vi "A14rowin.vi"(11 "Basic Size":ext) -> (3 "Row":ext)   [LabVIEW 2023]
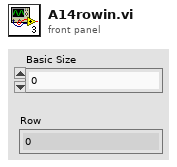
[diagram p1: front panel]
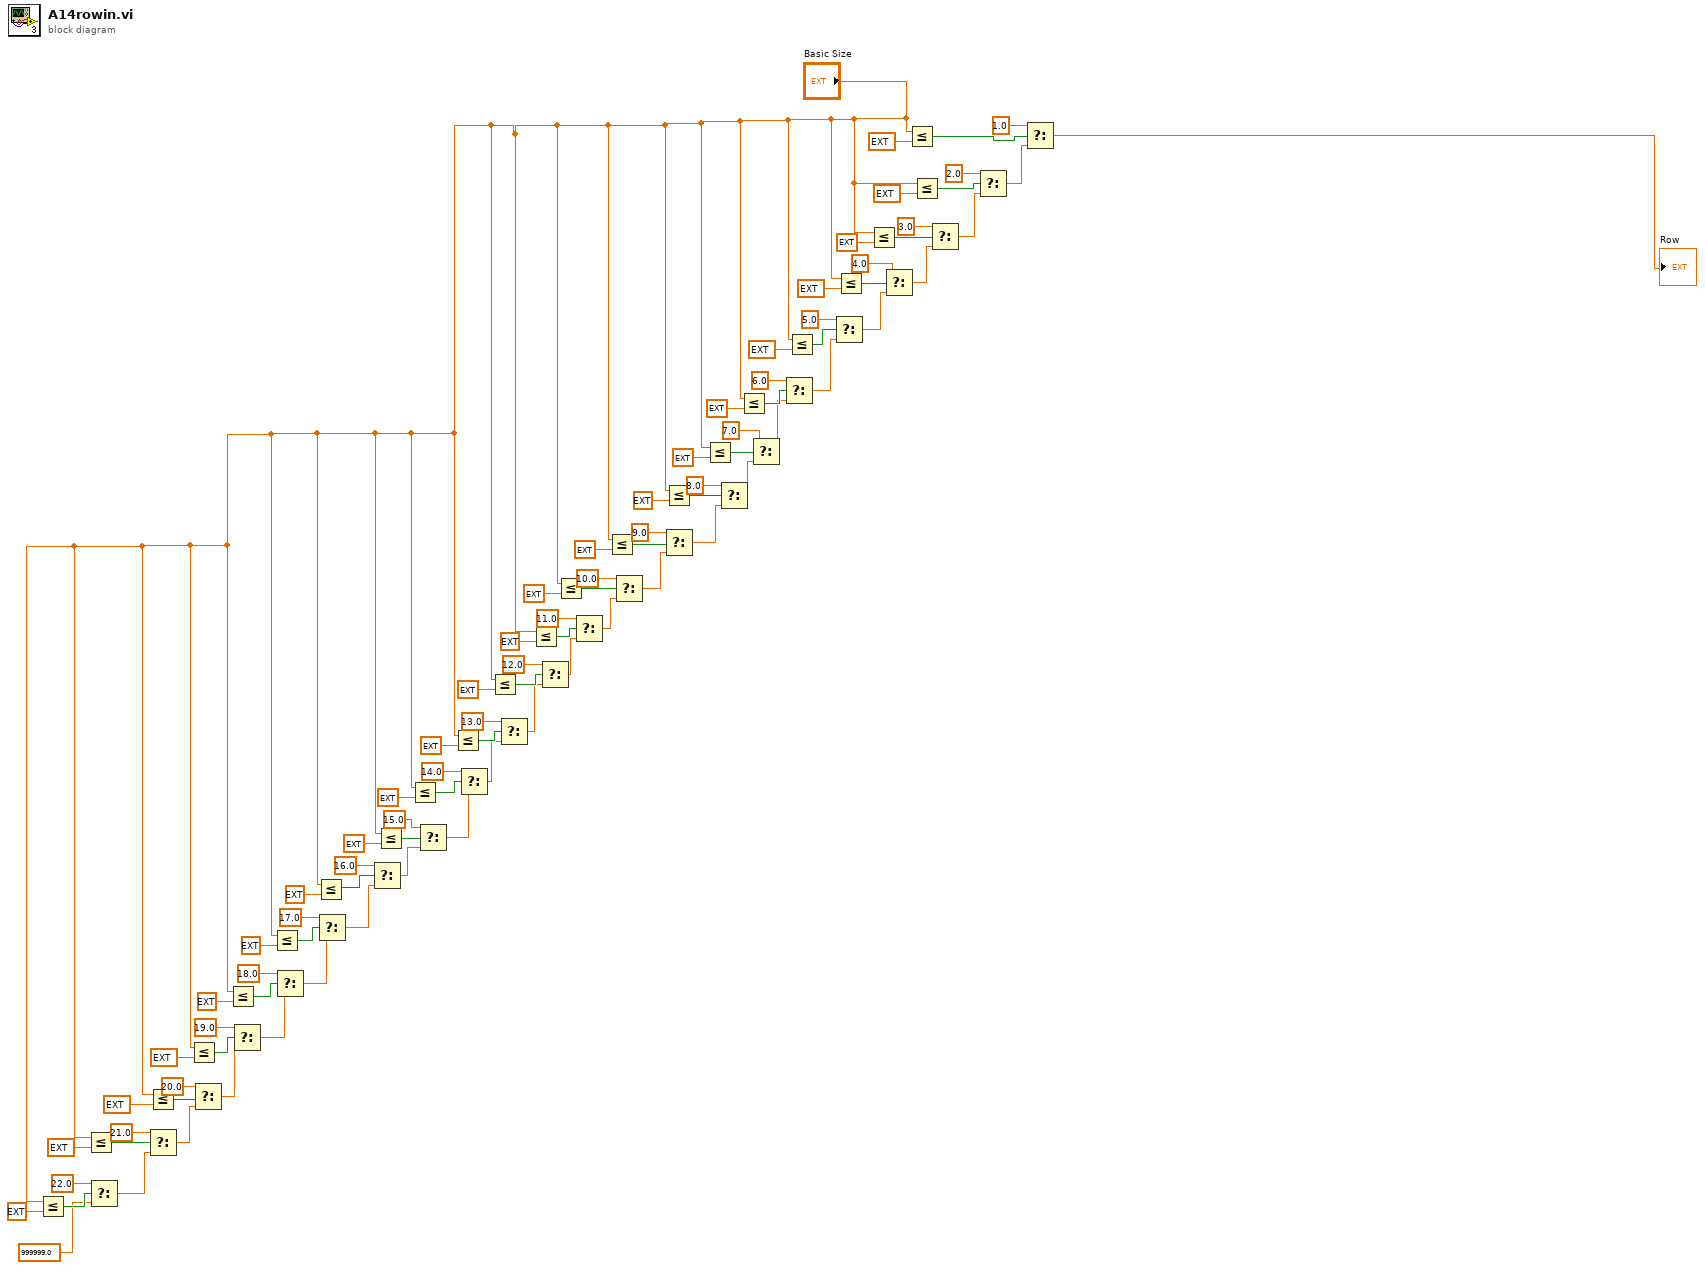
[diagram p0: block diagram]
diagram:
  n1 = Less Or Equal?(x="Basic Size", y=ext 16.0) -> (x <= y?=w4:bool)
  n2 = Less Or Equal?(x="Basic Size", y=ext 14.2) -> (x <= y?=w8:bool)
  n3 = Select(t=22.0, s=w4, f=999999.0) -> (s? t:f=w6:dbl)
  n4 = Less Or Equal?(x="Basic Size", y=ext 12.6000000000000000003) -> (x <= y?=w13:bool)
  n5 = Select(t=21.0, s=w8, f=w6) -> (s? t:f=w11:dbl)
  n6 = Less Or Equal?(x="Basic Size", y=ext 11.2) -> (x <= y?=w16:bool)
  n7 = Select(t=20.0, s=w13, f=w11) -> (s? t:f=w14:dbl)
  n8 = Less Or Equal?(x="Basic Size", y=ext 10.0) -> (x <= y?=w20:bool)
  n9 = Select(t=19.0, s=w16, f=w14) -> (s? t:f=w18:dbl)
  n10 = Less Or Equal?(x="Basic Size", y=ext 9.0) -> (x <= y?=w24:bool)
  n11 = Select(t=18.0, s=w20, f=w18) -> (s? t:f=w22:dbl)
  n12 = Less Or Equal?(x="Basic Size", y=ext 8.0) -> (x <= y?=w28:bool)
  n13 = Select(t=17.0, s=w24, f=w22) -> (s? t:f=w26:dbl)
  n14 = Select(t=16.0, s=w28, f=w26) -> (s? t:f=w30:dbl)
  n15 = Less Or Equal?(x="Basic Size", y=ext 7.2) -> (x <= y?=w32:bool)
  n16 = Less Or Equal?(x="Basic Size", y=ext 6.4) -> (x <= y?=w36:bool)
  n17 = Select(t=15.0, s=w32, f=w30) -> (s? t:f=w34:dbl)
  n18 = Less Or Equal?(x="Basic Size", y=ext 5.6) -> (x <= y?=w40:bool)
  n19 = Select(t=14.0, s=w36, f=w34) -> (s? t:f=w38:dbl)
  n20 = Less Or Equal?(x="Basic Size", y=ext 4.8000000000000000002) -> (x <= y?=w44:bool)
  n21 = Select(t=13.0, s=w40, f=w38) -> (s? t:f=w42:dbl)
  n22 = Less Or Equal?(x="Basic Size", y=ext 4.0) -> (x <= y?=w48:bool)
  n23 = Select(t=12.0, s=w44, f=w42) -> (s? t:f=w46:dbl)
  n24 = Less Or Equal?(x="Basic Size", y=ext 3.2) -> (x <= y?=w52:bool)
  n25 = Select(t=11.0, s=w48, f=w46) -> (s? t:f=w50:dbl)
  n26 = Less Or Equal?(x="Basic Size", y=ext 2.5999999999999999999) -> (x <= y?=w56:bool)
  n27 = Select(t=10.0, s=w52, f=w50) -> (s? t:f=w54:dbl)
  n28 = Less Or Equal?(x="Basic Size", y=ext 2.0) -> (x <= y?=w60:bool)
  n29 = Select(t=9.0, s=w56, f=w54) -> (s? t:f=w58:dbl)
  n30 = Less Or Equal?(x="Basic Size", y=ext 1.6) -> (x <= y?=w64:bool)
  n31 = Select(t=8.0, s=w60, f=w58) -> (s? t:f=w62:dbl)
  n32 = Less Or Equal?(x="Basic Size", y=ext 1.20000000000000000004) -> (x <= y?=w68:bool)
  n33 = Select(t=7.0, s=w64, f=w62) -> (s? t:f=w66:dbl)
  n34 = Select(t=6.0, s=w68, f=w66) -> (s? t:f=w70:dbl)
  n35 = Less Or Equal?(x="Basic Size", y=ext 0.96) -> (x <= y?=w72:bool)
  n36 = Select(t=5.0, s=w72, f=w70) -> (s? t:f=w74:dbl)
  n37 = Less Or Equal?(x="Basic Size", y=ext 0.72000000000000000003) -> (x <= y?=w77:bool)
  n38 = Less Or Equal?(x="Basic Size", y=ext 0.4) -> (x <= y?=w81:bool)
  n39 = Select(t=4.0, s=w77, f=w74) -> (s? t:f=w78:dbl)
  n40 = Less Or Equal?(x="Basic Size", y=ext 0.12) -> (x <= y?=w85:bool)
  n41 = Less Or Equal?(x="Basic Size", y=ext 0.24) -> (x <= y?=w84:bool)
  n42 = Select(t=3.0, s=w81, f=w78) -> (s? t:f=w82:dbl)
  n43 = Select(t=2.0, s=w84, f=w82) -> (s? t:f=w89:dbl)
  n44 = Select(t=1.0, s=w85, f=w89) -> (s? t:f=→"Row":dbl)
